vi "Chatper 3 Tank Value.vi"() -> ()   [LabVIEW 2018]
doc: "This VI is used to demonstrate the power of transparency."
panel:
  out "탱크 값":i32
  in  "불리언":bool
  in  "정지":bool
  out "탱크":i32(slide) scale=0.0..10.0
  # "값을 얻기 위해 탱크 값을 누르십시오."
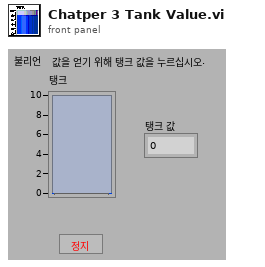
[diagram p1: front panel]
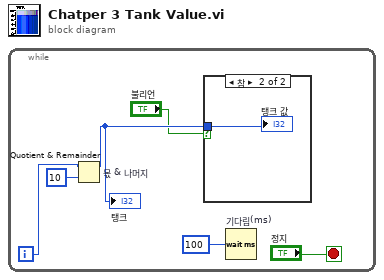
[diagram p0: block diagram]
diagram:
  n1 = while {
    i -> [w3]
    stop <- "정지" stop-if-true
    n2 = Quotient & Remainder "몫 & 나머지"(x=w3, y=10 ("floor(x/y)")) -> (x-y*floor(x/y)=w2:i32)  [unwired: 1 out]
    "탱크" <- w2
    n3 = case shown="참" "불리언" {
      tunnel: w2 -> [_ w7]
      frame False {
      }
      frame True {
        "탱크 값" <- w7
      }
    }
    n4 = Wait (ms) "기다림(ms)"(milliseconds to wait=u32 100) -> ()  [unwired: 1 out]
  }
